vi "GetCustomData.vi"(8 "error in":errorcluster, 11 "OperationRun in":refnum<class "OperationRun.lvclass">) -> (0 "error out":errorcluster, 2 "CustomData":refnum<class "CustomData.lvclass">, 3 "OperationRun out":refnum<class "OperationRun.lvclass">)   [LabVIEW 2021, in "ProligentXMLGenerator.lvlib" / "OperationRun.lvclass"]
doc: "Defines the name of the operation for this operation run.\n\nThis value must not be empty and is limited to 65 chars."
uses:
  OperationRun.lvclass
  OperationRun.lvclass/OperationRun.ctl
  Model/CustomData/CustomData.lvclass
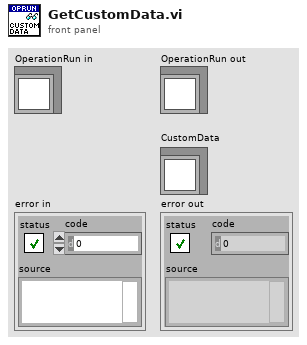
[diagram p1: front panel]
types:
  T1 = typedef "ProligentXMLGenerator.lvlib/OperationRun.lvclass/Data.ctl" = cluster{"Name":string, "Characteristics":refnum<class "Characteristic.lvclass">[], "Documents":refnum<class "Document.lvclass">[], "SequenceRuns":refnum<class "SequenceRun.lvclass">[], "FailureReferences":refnum<class "FailureReference.lvclass">[], "SequenceRunReferences":refnum<class "SequenceRunReference.lvclass">[], "CustomData":refnum<class "CustomData.lvclass">, "OperationRunId":refnum<class "Guid.lvclass">, "ProcessFullName":refnum<class "ProcessFullName.lvclass">, "ProcessVersion":refnum<class "NonEmptyString_64.lvclass">, "OperationName":refnum<class "NonEmptyString_65.lvclass">, "StationFullName":refnum<class "FullName.lvclass">, "User":refnum<class "NonEmptyString_255.lvclass">, "CallingOperationRunId":refnum<class "Guid.lvclass">, "OperationStatus":refnum<class "ExecutionStatus.lvclass">, "OperationRunStartTime":refnum<class "DateTime.lvclass">, "OperationRunEndTime":refnum<class "DateTime.lvclass">, "TimeZoneInfoId":string}
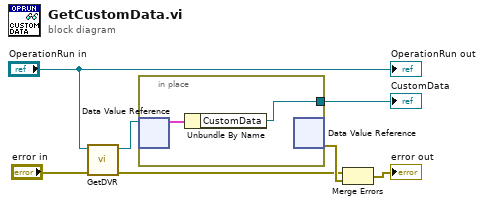
[diagram p0: block diagram]
diagram:
  n1 = call "GetDVR.vi"("error in"="error in", "OperationRun"="OperationRun in") -> ("error out"=w1:errorcluster, "DVRReference"=w6:refnum<data-value>)  [unwired: 8 in]
  n2 = in-place "In Place Element Structure" {
    in-place-border: [w8] -> w5
    n3 = in-place-dvr #1(w6) -> (w9:T1)  [unwired: 1 out]
    n4 = Unbundle By Name(w9) -> ("CustomData"=w8:refnum<class "CustomData.lvclass">)
    n5 = in-place-dvr #1() -> (w7:errorcluster)  [unwired: 1 in, 1 out]
  }
  "CustomData" <- w5
  n6 = Merge Errors(w1, w7) -> (→"error out":errorcluster)
  "OperationRun out" <- "OperationRun in"
